vi "ULx Write (Composite 1D Wfm NChan NSamp).vi"(0 "task in":refnum<k24>, 1 "auto start":bool, 5 "analog data":waveform(dbl)[](array[waveform]), 7 "digital data":digitalwaveform[](array[waveform]), 9 "timeout":dbl=10.0 format="%_4g", 11 "error in":errorcluster) -> (4 "task out":refnum<k24>, 10 "number of samples written per channel":u32, 15 "error out":errorcluster)   [LabVIEW 2020]
doc: "Writes one or more samples to a composite output task that contains that contains one or more analog output channels."
uses:
  C:/Users/William/Documents/LV 2020 builds/LeaktestDAQ/Source-v33/ULx_LV.dll
  ULx_LV.dll
  DWDT Digital Size.vi
  DTbl Digital to Binary U32.vi
panel:
  # "channel"
  # "channel"
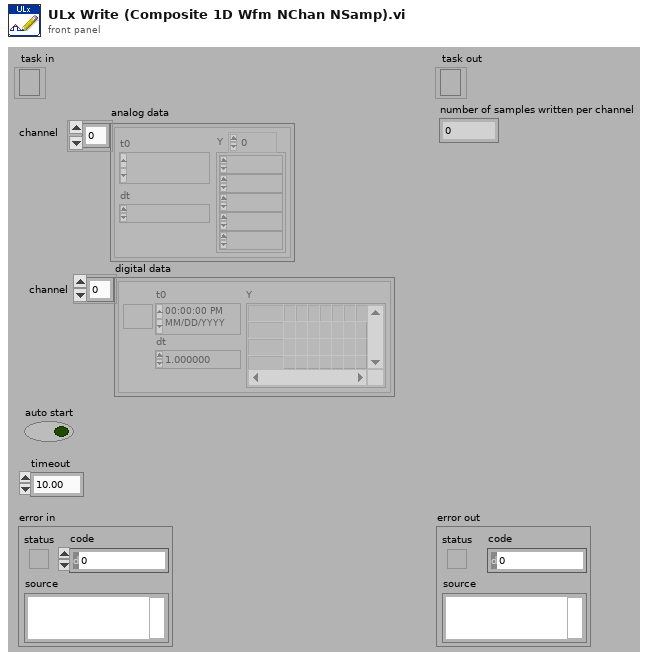
[diagram p1: front panel]
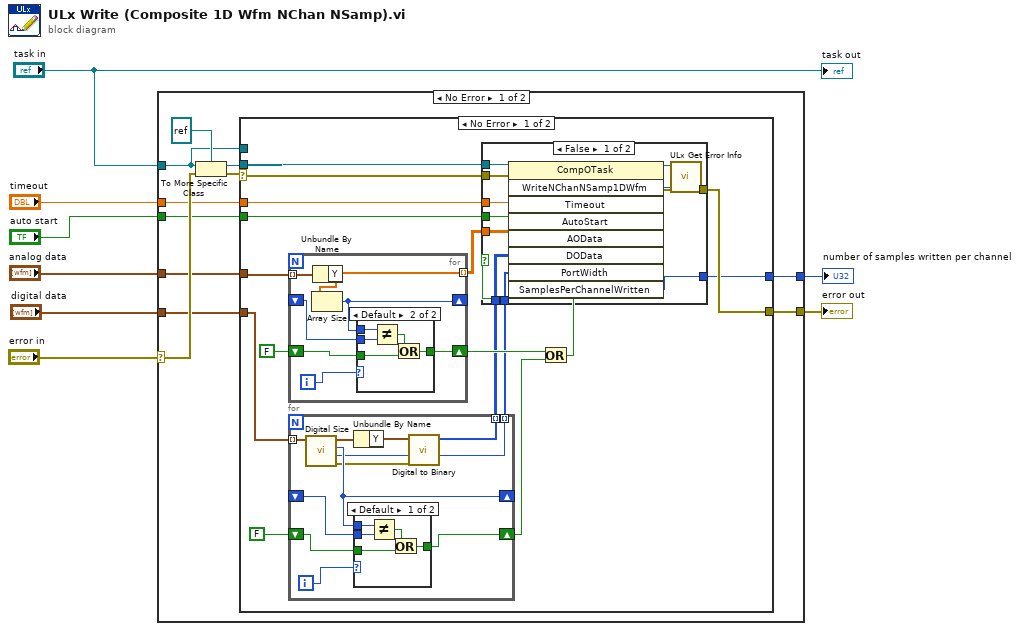
[diagram p0: block diagram]
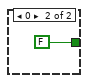
[diagram p2: hidden frame]
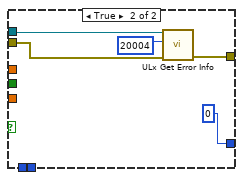
[diagram p3: hidden frame]
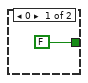
[diagram p4: hidden frame]
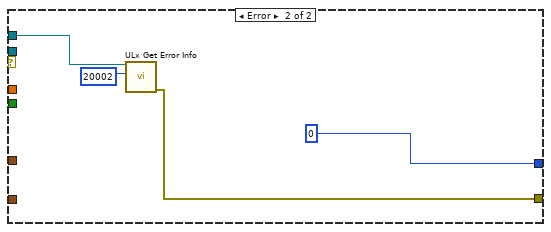
[diagram p5: hidden frame]
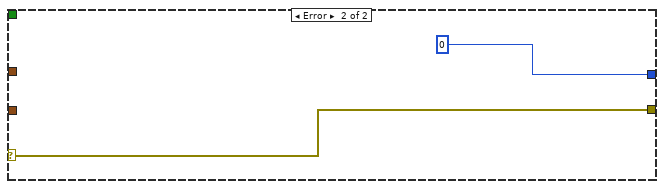
[diagram p6: hidden frame]
diagram:
  n1 = case shown="No Error" "error in" {
    selector: "error in" -> [w19 w88]
    tunnel: "task in" -> [w13 _]
    tunnel: "timeout" -> [w15 _]
    tunnel: [w14 w88] -> w6
    tunnel: "analog data" -> [w11 _]
    tunnel: "auto start" -> [w12 _]
    tunnel: [w10 0 ("SamplesPerChannelWritten")] -> w3
    tunnel: "digital data" -> [w9 _]
    frame No Error {
      n2 = To More Specific Class(target class=refnum<k24> refnum, reference=w13, error in=w19) -> (specific class reference=w16:refnum<k24>, error out=w17:errorcluster)
      n3 = case shown="No Error" w17 {
        selector: w17 -> [w34 _]
        tunnel: w16 -> [w35 _]
        tunnel: w15 -> [w32 _]
        tunnel: [w33 w85] -> w14
        tunnel: w13 -> [_ w84]
        tunnel: w12 -> [w31 _]
        tunnel: [w27 0 ("SamplesPerChannelWritten")] -> w10
        tunnel: w11 -> [w29 _]
        tunnel: w9 -> [w24 _]
        frame No Error {
          n4 = for {
            shift-right: [w75] -> _
            shift-left: _ -> [w74]
            tunnel: [w76] -> w30 mode=indexing
            tunnel: w29 -> [w73] mode=indexing
            shift-right: [w72] -> w26
            shift-left: FALSE -> [w71]
            i -> [w70]
            n5 = Unbundle By Name(w73) -> ("Y"=w76:dbl[])
            n6 = Array Size(array=w76) -> (size(s)=w75:i32)
            n7 = case shown="Default" w70 {
              tunnel: [FALSE w78] -> w72
              tunnel: w75 -> [_ w82]
              tunnel: w74 -> [_ w81]
              tunnel: w71 -> [_ w79]
              frame 0 {
              }
              frame Default {
                n8 = Not Equal?(x=w82, y=w81) -> (x != y?=w80:bool)
                n9 = Or(x=w80, y=w79) -> (x .or. y?=w78:bool)
              }
            }
          }
          n10 = for {
            tunnel: w24 -> [w46] mode=indexing
            shift-right: [w42] -> _
            shift-left: _ -> [w41]
            shift-right: [w40] -> w22
            shift-left: FALSE -> [w43]
            tunnel: [w38] -> w21 mode=indexing
            tunnel: [w37] -> w20 mode=indexing
            i -> [w36]
            n11 = call-poly "Digital Size.vi"("digital waveform in"=w46) -> ("error out"=w39:errorcluster, "number of signals"=w37:i32, "number of samples"=w42:i32, "digital waveform out"=w45:digitalwaveform)  [unwired: 7 in]
            n12 = Unbundle By Name(w45) -> ("Y"=w44:digitaldata)
            n13 = case shown="Default" w36 {
              tunnel: [w49 FALSE] -> w40
              tunnel: w43 -> [w50 _]
              tunnel: w42 -> [w48 _]
              tunnel: w41 -> [w47 _]
              frame Default {
                n14 = Not Equal?(x=w48, y=w47) -> (x != y?=w51:bool)
                n15 = Or(x=w51, y=w50) -> (x .or. y?=w49:bool)
              }
              frame 0 {
              }
            }
            n16 = call-poly "Digital to Binary.vi"("error in (no error)"=w39, "digital data"=w44) -> ("binary array"=w38:u32[])  [unwired: 8 in, 1 out]
          }
          n17 = Or(x=w26, y=w22) -> (x .or. y?=w25:bool)
          n18 = case shown="False" w25 {
            tunnel: w35 -> [w64 w66]
            tunnel: w34 -> [w63 w65]
            tunnel: [w60 w69] -> w33
            tunnel: [w53 u32 0 ("SamplesPerChannelWritten")] -> w27
            tunnel: w32 -> [w58 _]
            tunnel: w31 -> [w57 _]
            tunnel: w30 -> [w56 _]
            tunnel: w21 -> [w55 _]
            tunnel: w20 -> [w54 _]
            frame False {
              n19 = invoke class="CompOTask" method="WriteNChanNSamp1DWfm"(reference=w64, error in=w63, "Timeout"=w58, "AutoStart"=w57, "AOData"=w56, "DOData"=w55, "PortWidth"=w54) -> (reference out=w61:refnum<k24>, error out=w62:errorcluster, "WriteNChanNSamp1DWfm"=w59:i32, "SamplesPerChannelWritten"=w53:u32)  [unwired: 2 in, 5 out]
              n20 = call "ULx Get Error Info.vi"("error in"=w62, "ErrorCode"=w59, "task in"=w61) -> ("error out"=w60:errorcluster)  [unwired: 8 in]
            }
            frame True {
              n21 = call "ULx Get Error Info.vi"("error in"=w65, "ErrorCode"=20004, "task in"=w66) -> ("error out"=w69:errorcluster)  [unwired: 8 in]
            }
          }
        }
        frame Error {
          n22 = call "ULx Get Error Info.vi"("ErrorCode"=20002, "task in"=w84) -> ("error out"=w85:errorcluster)  [unwired: 9 in]
        }
      }
    }
    frame Error {
    }
  }
  "error out" <- w6
  "number of samples written per channel" <- w3
  "task out" <- "task in"
